vi "Potting Data - HV Points.vi"(10 "HV Point Selection":bool[](array[boolean]), 11 "HV Point Data":T1[](array[typedef])) -> (3 "HV Potting Points":refnum<class "Vec3d Class.lvclass">[](array[class]))   [LabVIEW 2011]
uses:
  Shared Components/Vec3d Class/Vec3d Class.lvclass
  Shared Components/Utils/Type Definitions/Fiducial Image.ctl
  Shared Components/Utils/Type Definitions/Physical Image.ctl
  <vilib>/vision/Image Controls.llb/IMAQ Image.ctl
  Shared Components/Utils/Type Definitions/Fiducial with Source.ctl
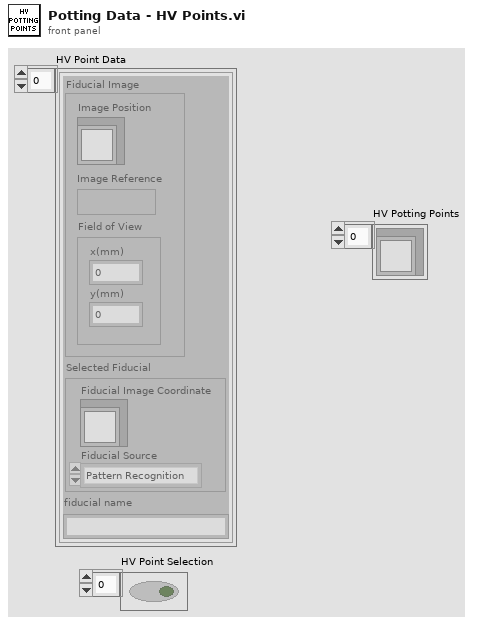
[diagram p1: front panel]
types:
  T1 = typedef "Fiducial Image.ctl" = cluster{"Fiducial Image":T2, "Selected Fiducial":T4, "fiducial name":string}
  T2 = typedef "Physical Image.ctl" = cluster{"Image Position":refnum<class "Vec3d Class.lvclass">, "Image Reference":T3, "Field of View":cluster{"x(mm)":dbl, "y(mm)":dbl}}
  T3 = typedef "IMAQ Image.ctl" = refnum<image>
  T4 = typedef "Fiducial with Source.ctl" = cluster{"Fiducial Image Coordinate":refnum<class "Vec3d Class.lvclass">, "Fiducial Source":enum16{"Pattern Recognition", "User", "Error", "Default"}}
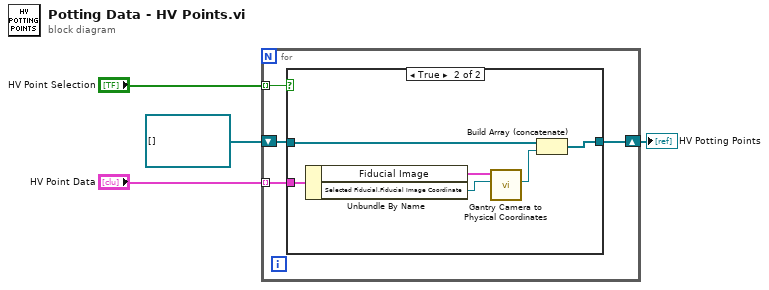
[diagram p0: block diagram]
diagram:
  n1 = for {
    tunnel: "HV Point Data" -> [w6] mode=indexing
    tunnel: "HV Point Selection" -> [w7] mode=indexing
    shift-right: [w5] -> w3
    shift-left: refnum<class "Vec3d Class.lvclass">[] [] ("appended array") -> [w8]
    n2 = case shown="True" w7 {
      tunnel: w8 -> [w9 w15]
      tunnel: w6 -> [_ w13]
      tunnel: [w9 w14] -> w5
      frame False {
      }
      frame True {
        n3 = Unbundle By Name(w13) -> ("Fiducial Image"=w12:T2, "Selected Fiducial.Fiducial Image Coordinate"=w11:refnum<class "Vec3d Class.lvclass">)
        n4 = call "Gantry Camera to Physical Coordinates.vi"("Image Coordinate"=w11, "Physical Image"=w12) -> ("Global Coordinate"=w10:refnum<class "Vec3d Class.lvclass">)  [unwired: 7 in, 2 out]
        n5 = Build Array (concatenate)(w15, w10) -> (w14:refnum<class "Vec3d Class.lvclass">[])
      }
    }
  }
  "HV Potting Points" <- w3
